vi "Clousure.vi"(8 "error in (no error)":errorcluster, 11 "PizzaStore":refnum<class "PizzaStore.lvclass">) -> (0 "error out":errorcluster, 3 "PizzaStore":refnum<class "PizzaStore.lvclass">)   [LabVIEW 2020, in "FactoryMethod.lvlib" / "PizzaFactoryMethod.lvlib" / "PizzaStore.lvclass"]
uses:
  PizzaStore.lvclass
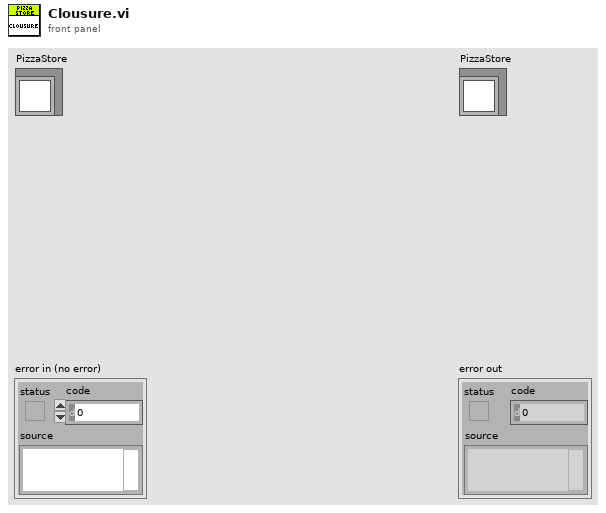
[diagram p1: front panel]
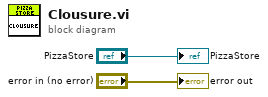
[diagram p0: block diagram]
diagram:
  "error out" <- "error in (no error)"
  "PizzaStore" <- "PizzaStore"
